vi "daq_pressure_sensors.vi"(1 "Timeout":i32) -> (0 "FIFO_timeout":bool)   [LabVIEW 2018]
uses:
  <vilib>/rvi/eio/common/nirviEmuTemplateMethod_errors.vi
  <vilib>/rvi/DataTransferAndStorage/Container/Common/niFpgaContainerExecOnDevCompGetState.vi
  <vilib>/rvi/Emulation/niFpgaEmulationIsFPGAContextNoSignature.vi
  <vilib>/rvi/Emulation/niFpgaSctlEmulationGetInTimedLoop.vi
  <vilib>/rvi/errors/niFpgaSetErrorForExecOnDevCompSimple.vi
  <vilib>/rvi/eio/common/nirviEmuReportErrorAndStop.vi
  <vilib>/rvi/DataTransferAndStorage/Container/Common/niFpgaContainerGetUniqueNameForEmu.vi
  <vilib>/rvi/FIFO/Fifo_Resource/nirvififoEmulationSetSize.vi
  <vilib>/rvi/FIFO/Fifo_Resource/nirviFifoEmulationQueueMgr.vi
  <instcachedir>/0/nirviFifoEmulationQueueMgr_E5CAEC123FF24DC58D834DCA3CDAA9B5.lvgen/nirviFifoEmulationQueueMgr_E5CAEC123FF24DC58D834DCA3CDAA9B5_002.vi
  <vilib>/rvi/FIFO/Fifo_Resource/nirvififoEmulationDetermineInputValidOut.vi
  <vilib>/rvi/FIFO/Fifo_Resource/nirvififoEmulationCreateLock.vi
  <vilib>/rvi/Emulation/niFpgaProcessEmulError.vi
  <vilib>/rvi/FIFO/Fifo_Resource/nirvififoEmulationObtainLock.vi
  <vilib>/rvi/FIFO/Fifo_Resource/nirvififoEmulationReleaseLock.vi
  <vilib>/rvi/occurrence/nirviWaitOnOccurrenceBase.vi
  <vilib>/rvi/errors/nirviReportUnexpectedCaseInternalError.vi
  <vilib>/rvi/errors/nirviReportUnexpectedCaseInternalError (U32).vi
  <vilib>/Utility/error.llb/Clear Errors.vi
  <vilib>/rvi/interface/RandomDataEmulation/niFpgaRandomDataHandleErrors.vi
  <vilib>/eio/EIONode/EIONode.xnode
  <vilib>/rvi/DataTransferAndStorage/Container/XNode/niFpgaContainer.xnode
  <vilib>/rvi/FIFO/Fifo_Resource/niFpgaFifoEmulationRefIn.vi
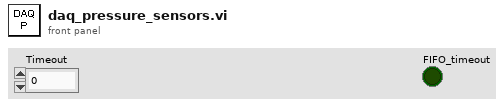
[diagram p1: front panel]
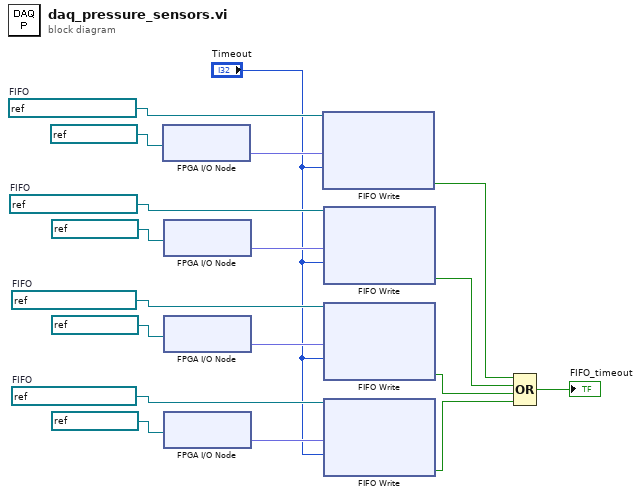
[diagram p0: block diagram]
diagram:
  w8 = refnum<k21> "P_transducer_LP_2"  # FIFO
  w11 = refnum<k21> "P_transducer_LP_1"  # FIFO
  w14 = refnum<k21> "P_transducer_HP_2"  # FIFO
  w17 = refnum<k21> "P_transducer_HP_1"  # FIFO
  n1 = xnode "FPGA I/O Node"("FPGA I/O In"=refnum<k21> "Mod1/AI14") -> ("I/O Item"=w16:fxp<+/-,24,5>)  [unwired: 1 out]
  n2 = xnode "FPGA I/O Node"("FPGA I/O In"=refnum<k21> "Mod1/AI15") -> ("I/O Item"=w13:fxp<+/-,24,5>)  [unwired: 1 out]
  n3 = xnode "FPGA I/O Node"("FPGA I/O In"=refnum<k21> "Mod1/AI16") -> ("I/O Item"=w10:fxp<+/-,24,5>)  [unwired: 1 out]
  n4 = xnode "FPGA I/O Node"("FPGA I/O In"=refnum<k21> "Mod1/AI17") -> ("I/O Item"=w7:fxp<+/-,24,5>)  [unwired: 1 out]
  n5 = xnode "FIFO Write"("Element"=w16, "Timeout"="Timeout", "FIFO In"=w17) -> ("Timed Out?"=w5:bool)  [unwired: 1 out]
  n6 = xnode "FIFO Write"("Element"=w13, "Timeout"="Timeout", "FIFO In"=w14) -> ("Timed Out?"=w4:bool)  [unwired: 1 out]
  n7 = xnode "FIFO Write"("Element"=w10, "Timeout"="Timeout", "FIFO In"=w11) -> ("Timed Out?"=w3:bool)  [unwired: 1 out]
  n8 = xnode "FIFO Write"("Element"=w7, "Timeout"="Timeout", "FIFO In"=w8) -> ("Timed Out?"=w2:bool)  [unwired: 1 out]
  n9 = Compound Arithmetic op=OR(w5, w4, w3, w2) -> (→"FIFO_timeout":bool)
